vi "Get date and time stub for end of file.vi"() -> (0 "date and time stub":string="_2007Y_10M_02D_21h_06m_40s")   [LabVIEW 2015]
panel:
  out "second":string="40"
  out "minute":string="06"
  out "hour":string="21"
  out "day":string="02"
  out "month":string="10"
  out "year":string="2007"
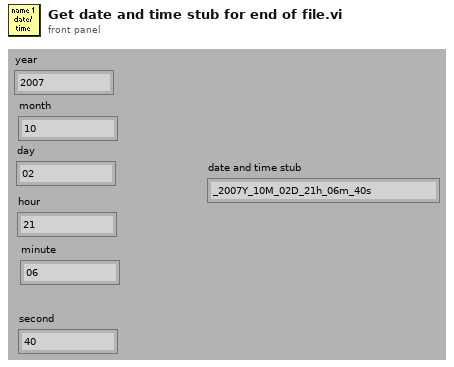
[diagram p1: front panel]
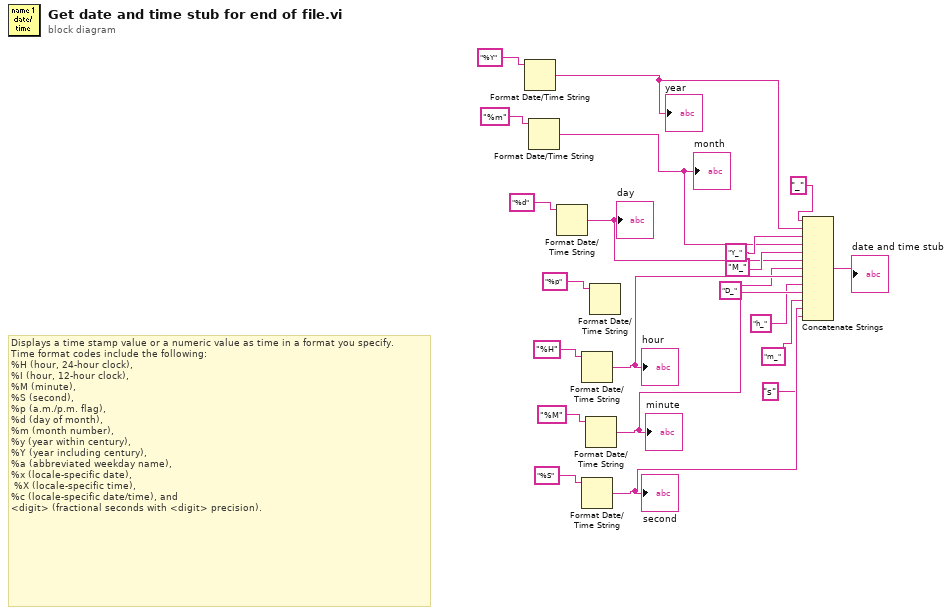
[diagram p0: block diagram]
diagram:
  # "Displays a time stamp value or a numeric value as time in a format you specify. \nTime format codes include the following: \n%H (hour, 24-hour clock), \n%I (hour, 12-hour clock), \n%M (minute), \n%S (second), \n%p (a.m./p.m. flag), \n%d (day of month),\n%m (month number), \n%y (year within century), \n%Y (year including century),\n%a (abbreviated weekday name), \n%x (locale-specific date),\n %X (locale-specific time), \n%c (locale-specific date/time), and \n<digit> (fractional seconds with <digit> precision)."
  n1 = Format Date/Time String(time format string (%c)="%Y") -> (date/time string=w5:string)  [unwired: 2 out]
  "year" <- w5
  n2 = Format Date/Time String(time format string (%c)="%m") -> (date/time string=w4:string)  [unwired: 2 out]
  "month" <- w4
  n3 = Format Date/Time String(time format string (%c)="%d") -> (date/time string=w3:string)  [unwired: 2 out]
  "day" <- w3
  n4 = Format Date/Time String(time format string (%c)="%H") -> (date/time string=w11:string)  [unwired: 2 out]
  "hour" <- w11
  n5 = Format Date/Time String(time format string (%c)="%S") -> (date/time string=w13:string)  [unwired: 2 out]
  "second" <- w13
  n6 = Format Date/Time String(time format string (%c)="%M") -> (date/time string=w14:string)  [unwired: 2 out]
  "minute" <- w14
  n7 = Format Date/Time String(time format string (%c)="%p") -> ()  [unwired: 3 out]
  n8 = Concatenate Strings("_", w5, "Y_", w4, "M_", w3, "D_", w11, "h_", w14, "m_", w13, "s") -> (→"date and time stub":string)
